vi "snr_real_test.vi"() -> ()   [LabVIEW 2020]
uses:
  <vilib>/Waveform/WDTOps.llb/WDT Get Waveform Subset DBL.vi
panel:
  in  "resultant?":bool=TRUE
  out "time":waveform(dbl)(graph)
  in  "reset cursor":bool
  in  "sec":dbl=30.0 format="%#_13g"
  out "Waveform Graph":waveform(dbl)[](graph)
  in  "start":timestamp
  in  "invert?":bool
  in  "acc?":bool=TRUE
  in  "axis":i32
  out "Csapásszám [stroke/min]":dbl
  in  "file path (use dialog)":path
  in  "felharmonikus N":i32
  out "kiolvasott frekvencia [Hz]":dbl
  out "Noise Integral":dbl
  out "Signal Integral":dbl
  out "SNR":dbl
  out "PSD":cluster{"f0":dbl, "df":dbl, "magnitude":dbl[]}[](graph)
  in  "ablak szélesség [Hz]":dbl=0.2 format="%#_13g"
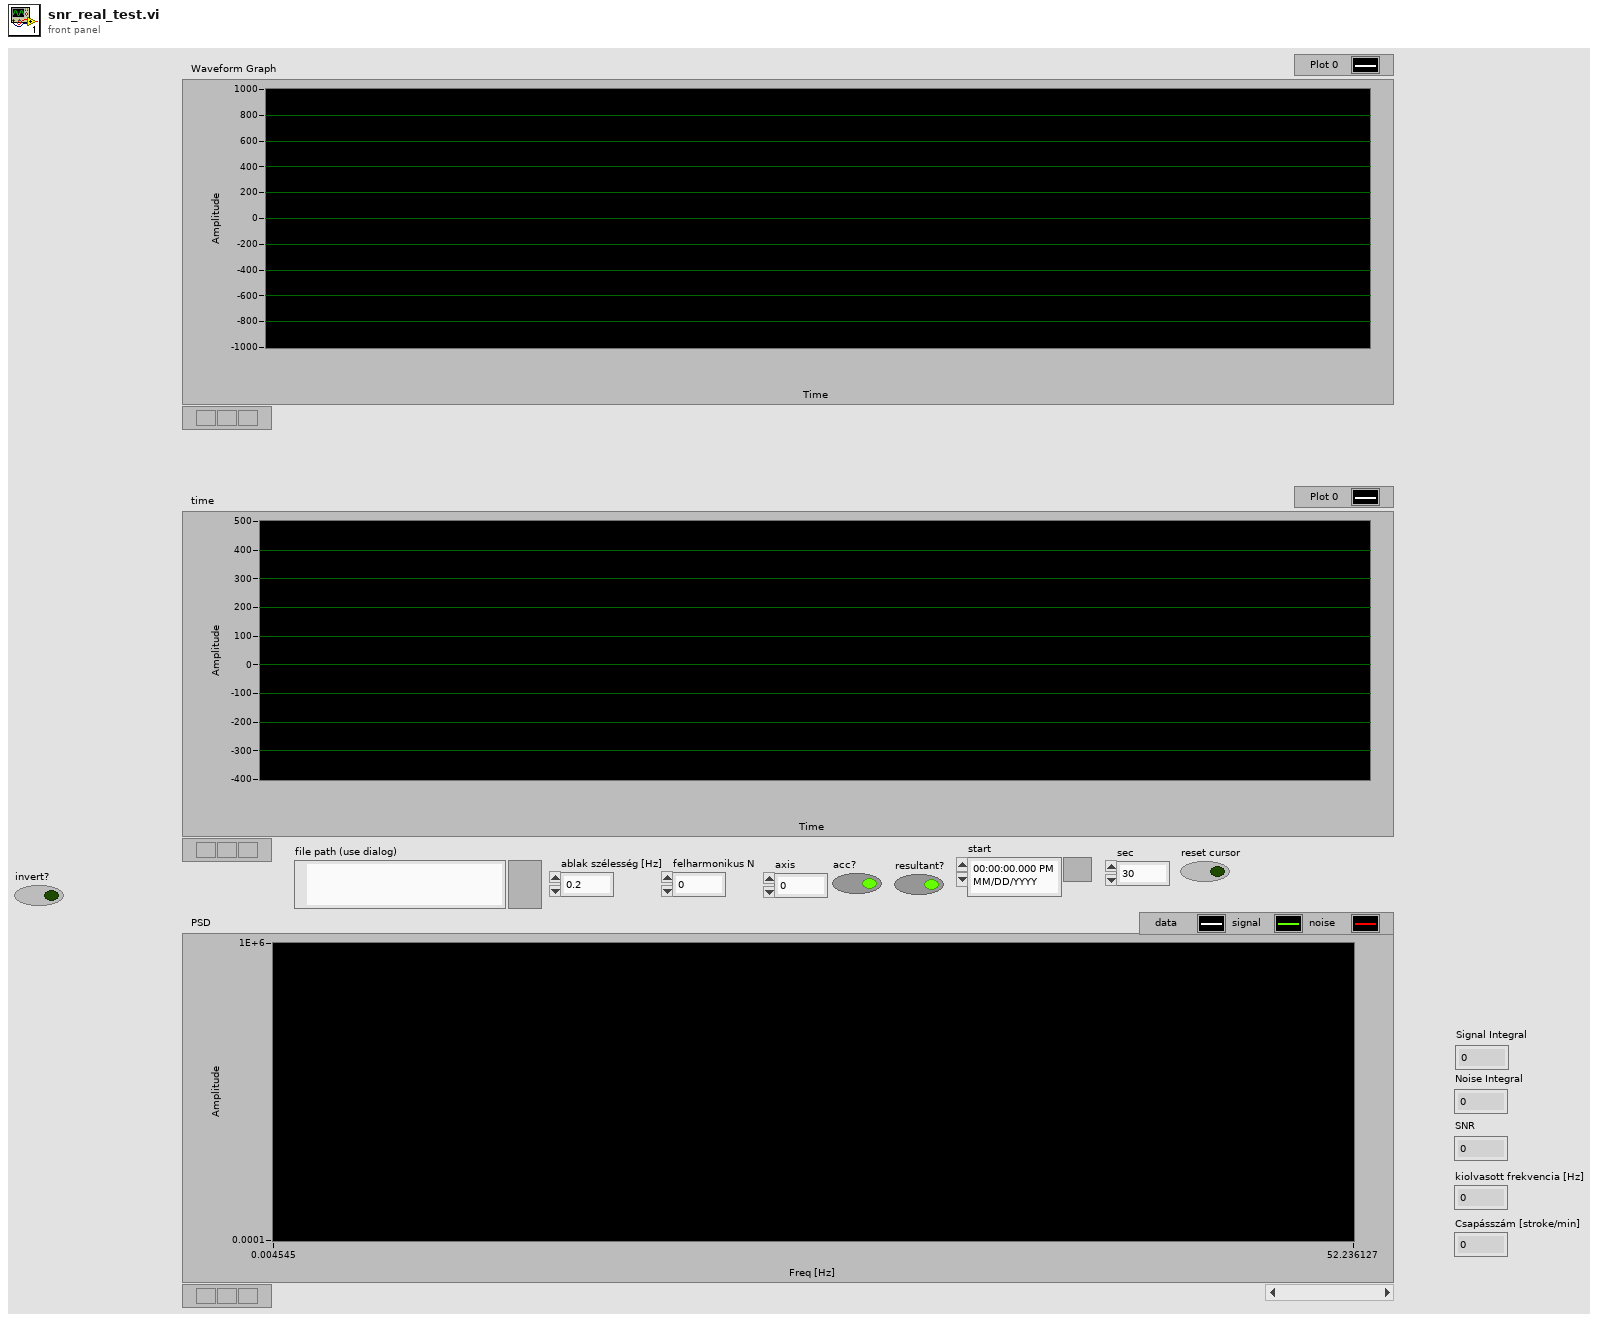
[diagram p1: front panel]
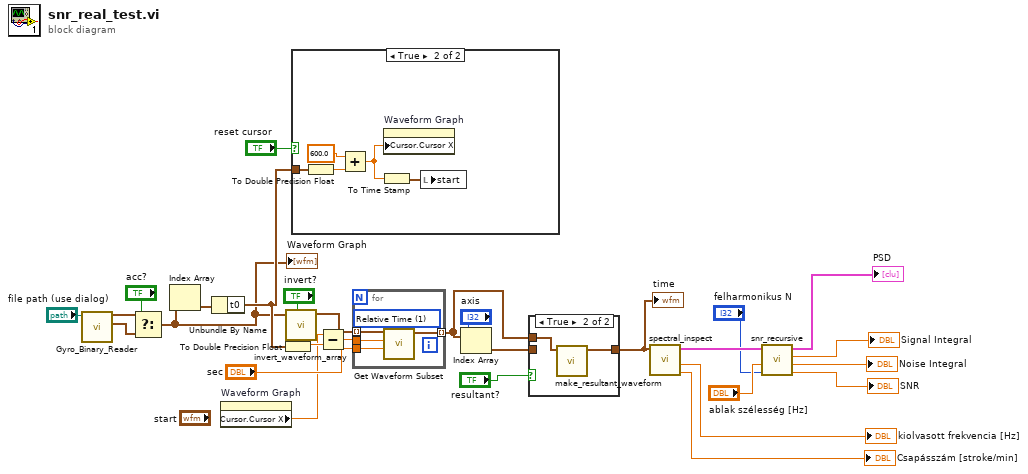
[diagram p0: block diagram]
diagram:
  n1 = call "Gyro_Binary_Reader.vi"("file path (use dialog)"="file path (use dialog)") -> ("Angular Velocity"=w13:waveform(dbl)[], "Acceleration"=w14:waveform(dbl)[])  [unwired: 7 in, 2 out]
  n2 = Select(t=w14, s="acc?", f=w13) -> (s? t:f=w5:waveform(dbl)[])
  "Waveform Graph" <- w5
  n3 = Index Array(array=w5) -> (element=w9:waveform(dbl))  [unwired: 1 in]
  n4 = Unbundle By Name(w9) -> ("t0"=w6:timestamp)
  n5 = property on="Waveform Graph" class="WFGraph (strict)"() -> ("Cursor.Cursor X"=w7:dbl)  [unwired: 2 in, 2 out]
  n6 = To Double Precision Float(number=w6) -> (double precision float=w17:dbl)
  n7 = call "invert_waveform_array.vi"("Invert x"="invert?", "x, y, z axis data"=w5) -> ("inverted x waveform array"=w16:waveform(dbl)[])  [unwired: 9 in]
  n8 = case shown="True" "reset cursor" {
    tunnel: w6 -> [_ w33]
    frame False {
    }
    frame True {
      n9 = To Double Precision Float(number=w33) -> (double precision float=w32:dbl)
      n10 = Add(x=600.0, y=w32) -> (x+y=w29:dbl)
      n11 = To Time Stamp(1:w29) -> (0:w30:timestamp)
      n12 = property on="Waveform Graph" class="WFGraph (strict)"("Cursor.Cursor X"=w29) -> ()  [unwired: 2 in, 2 out]
      n13 = local write "start"(w30) -> ()
    }
  }
  n14 = Subtract(x=w7, y=w17) -> (x-y=w18:dbl)
  n15 = for {
    tunnel: w16 -> [w38] mode=indexing
    tunnel: [w37] -> w1 mode=indexing
    tunnel: "sec" -> [w36]
    tunnel: w18 -> [w35]
    w34 = u16 1 items=["Samples", "Relative Time"] ("start/duration format")
    n16 = call-poly <vilib>:"Get Waveform Subset.vi"("start/duration format"=w34, "duration"=w36, "start samples/time"=w35, "waveform in"=w38) -> ("waveform out"=w37:waveform(dbl))  [unwired: 2 in, 3 out]
  }
  n17 = Index Array(array=w1, index="axis") -> (element=w4:waveform(dbl))
  n18 = case shown="True" "resultant?" {
    tunnel: w4 -> [w39 _]
    tunnel: [w39 w41] -> w3
    tunnel: w1 -> [_ w40]
    frame False {
    }
    frame True {
      n19 = call "make_resultant_waveform.vi"("waveform array"=w40) -> ("inspected resultant"=w41:waveform(dbl))  [unwired: 9 in, 1 out]
    }
  }
  "time" <- w3
  n20 = call "spectral_inspect.vi"("waveform"=w3) -> ("Csapásszám [stroke/min]"=→"Csapásszám [stroke/min]":dbl, "freq"=→"kiolvasott frekvencia [Hz]":dbl, "PSD"=w28:cluster{"f0":dbl, "df":dbl, "magnitude":dbl[]})  [unwired: 6 in, 2 out]
  n21 = call "snr_recursive.vi"("felharmonikus N"="felharmonikus N", "width [Hz]"="ablak szélesség [Hz]", "PSD"=w28) -> ("SNR"=→"SNR":dbl, "Noise Integral"=→"Noise Integral":dbl, "Signal Integral"=→"Signal Integral":dbl, "PSD"=→"PSD":cluster{"f0":dbl, "df":dbl, "magnitude":dbl[]}[])  [unwired: 5 in]
